vi "DashboardIsProgramSaved.vi"(8 "Dashboard":refnum<k24>, 11 "error in":errorcluster) -> (0 "Response":cluster{"Message":string, "Succeed":bool}, 1 "IsSaved":bool, 2 "Name":string, 3 "error out":errorcluster)   [LabVIEW 2023, in "UnderAutomation.UniversalRobots.lvlib"]
uses:
  UnderAutomation.UniversalRobots.lvlib
  C:/Users/fg/Documents/UniversalRobots.vi/UnderAutomation.UniversalRobots/lib/UnderAutomation.UniversalRobots.dll
  lib/UnderAutomation.UniversalRobots.dll
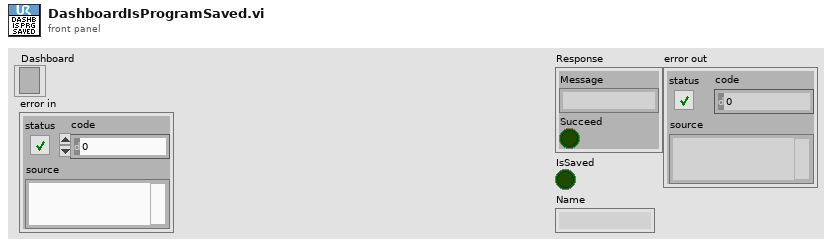
[diagram p1: front panel]
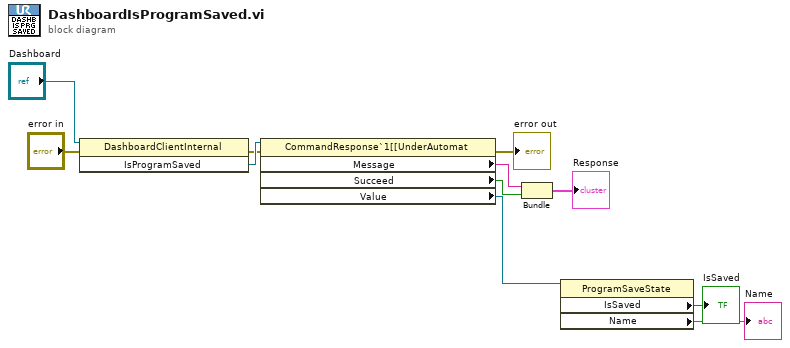
[diagram p0: block diagram]
diagram:
  n1 = invoke class="DashboardClientInternal" method="IsProgramSaved"(reference="Dashboard", error in="error in") -> (error out=w5:errorcluster, "IsProgramSaved"=w10:refnum<k24>)  [unwired: 1 in, 1 out]
  n2 = property class="CommandResponse`1[[UnderAutomat"(reference=w10, error in=w5) -> (error out=→"error out":errorcluster, "Message"=w9:string, "Succeed"=w8:bool, "Value"=w3:refnum<k24>)  [unwired: 1 out]
  n3 = Bundle("Message"=w9, "Succeed"=w8) -> (→"Response":cluster{"Message":string, "Succeed":bool})  [unwired: 1 in]
  n4 = property class="ProgramSaveState"(reference=w3) -> ("IsSaved"=→"IsSaved":bool, "Name"=→"Name":string)  [unwired: 1 in, 2 out]
